vi "Constant - Default Sample Rate (Hz).vi"() -> (3 "Streaming Rate (Hz)":i32=10)   [LabVIEW 2021]
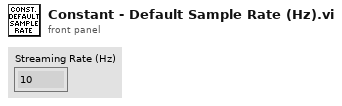
[diagram p1: front panel]
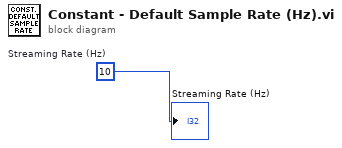
[diagram p0: block diagram]
diagram:
  w1 = 10  # Streaming Rate (Hz)
  "Streaming Rate (Hz)" <- w1
